vi "proje ödevi.vi"() -> ()   [LabVIEW 2017]
uses:
  <vilib>/MakerHub/LINX/Public/Peripherals/Analog/Analog Read 1 Chan.vi
  <vilib>/MakerHub/LINX/Public/Peripherals/Digital/Digital Write 1 Chan.vi
  <vilib>/MakerHub/LINX/Public/Peripherals/Analog/Analog Read N Chans.vi
  <vilib>/MakerHub/LINX/Public/Peripherals/Digital/Digital Write N Chans.vi
  <vilib>/MakerHub/LINX/Private/Local IO/LinxAnalogRead.vi
  <vilib>/MakerHub/LINX/Public/Utilities/Check Channel.vi
  <vilib>/MakerHub/LINX/Private/Local IO/LinxDigitalWrite.vi
  <vilib>/MakerHub/LINX/Public/Utilities/Open Serial.vi
  <vilib>/MakerHub/LINX/Private/Utilties/Generate Error.vi
  <vilib>/MakerHub/LINX/LMH-LINX.lvlib
panel:
  in  "Soğutucu çalıştırma değeri":dbl=29.0
  in  "Isıtıcı çalıştırma değeri":dbl=24.0
  in  "?":refnum<visa-resource-name>="COM3"
  out "Termometre":dbl(slide) scale=0.0..100.0
  out "?":dbl
  out "Voltage":dbl
  in  "?":bool
  # "Bağlantı İşlemleri"
  # "Sıcaklık Ayarı"
  # "Gösterge Paneli"
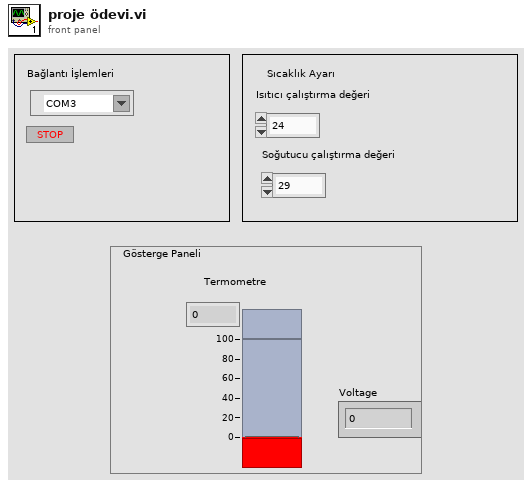
[diagram p1: front panel]
types:
  T1 = typedef "LMH-LINX.lvlib/LINX Ref.ctl" = cluster{"IO":T2, "Interface":T3, "LINX Device Config":T4}
  T2 = typedef "LMH-LINX.lvlib/Platform.ctl" = enum16{"Remote", "Local"}
  T3 = typedef "LMH-LINX.lvlib/Interface.ctl" = enum16{"Serial", "TCP"}
  T4 = typedef "LMH-LINX.lvlib/Device.lvlib/LINX Device Config.ctl" = cluster{"Interface":T3, "COM Port":refnum<visa-resource-name>, "TCP Configuration":T5, "Device Family":u8, "Device ID":u8, "Device Name":string, "TCP Ref":refnum<k5>, "Channels":T6}
  T5 = typedef "LMH-LINX.lvlib/Device.lvlib/TCP Config.ctl" = cluster{"IP Address":string, "Port":u16}
  T6 = typedef "LMH-LINX.lvlib/Channels.ctl" = cluster{"DI":u8[], "DO":u8[], "AI":u8[], "AO":u8[], "PWM":u8[], "QE":u8[], "UART":u8[], "I2C 2":u8[], "SPI":u8[], "CAN":u8[], "Servo":u8[], "AI Ref (V)":dbl, "AI Resolution (Bits)":u8, "AO Ref (V)":dbl, "AO Resolution (Bits)":u8}
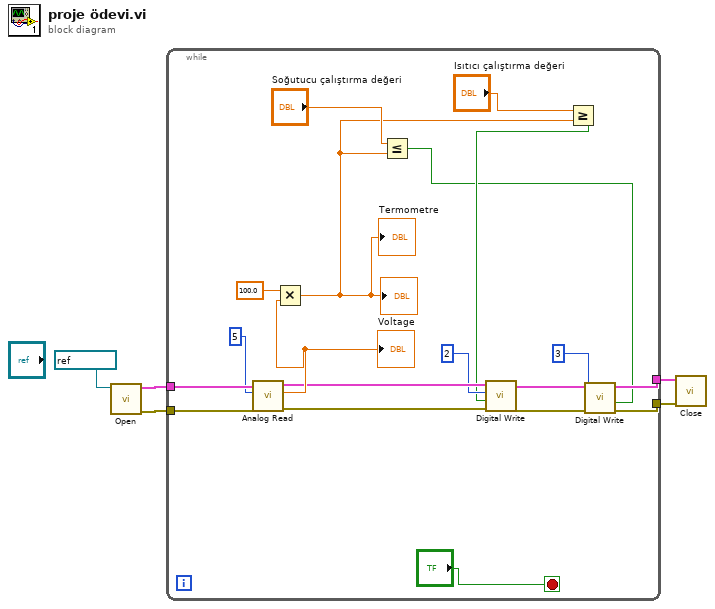
[diagram p0: block diagram]
diagram:
  n1 = call-poly <vilib>:"Open.vi"("Serial Port"=refnum<visa-resource-name> "COM3") -> ("Error Out"=w4:errorcluster, "LINX Resource"=w3:T1)  [unwired: 8 in, 1 out]
  n2 = while {
    tunnel: w4 -> [w24]
    tunnel: w3 -> [w23]
    tunnel: [w12] -> w2
    tunnel: [w11] -> w1
    stop <- "?" stop-if-true
    n3 = call-poly <vilib>:"Analog Read.vi"("Error In"=w24, "Analog Channel"=u8 5, "LINX Resource"=w23) -> ("Error Out"=w17:errorcluster, "Voltage"=w19:dbl, "LINX Resource"=w18:T1)  [unwired: 5 in, 1 out]
    "Voltage" <- w19
    n4 = Multiply(x=100.0, y=w19) -> (x*y=w6:dbl)
    "?" <- w6
    "Termometre" <- w6
    n5 = Less Or Equal?(x="Soğutucu çalıştırma değeri", y=w6) -> (x <= y?=w9:bool)
    n6 = Greater Or Equal?(x="Isıtıcı çalıştırma değeri", y=w6) -> (x >= y?=w15:bool)
    n7 = call-poly <vilib>:"Digital Write.vi"("Error In"=w17, "Output Value"=w15, "DO Channel"=u8 2, "LINX Resource"=w18) -> ("Error Out"=w13:errorcluster, "LINX Resource"=w14:T1)  [unwired: 6 in]
    n8 = call-poly <vilib>:"Digital Write.vi"("Error In"=w13, "Output Value"=w9, "DO Channel"=u8 3, "LINX Resource"=w14) -> ("Error Out"=w12:errorcluster, "LINX Resource"=w11:T1)  [unwired: 6 in]
  }
  n9 = call <vilib>:"Close.vi"("Error In"=w2, "LINX Resource"=w1) -> ()  [unwired: 9 in, 1 out]
